vi "unpackAutonArray.vi"(0 "all rows":dbl[][](array[numeric])) -> (19 "ShootNow":dbl[](array[numeric]), 20 "Primitive":i16[](array[numeric]), 21 "Left Drive":dbl[](array[numeric]), 22 "Right Drive":dbl[](array[numeric]), 23 "Ramp ACT":dbl[](array[numeric]), 24 "Conveyor":dbl[](array[numeric]), 25 "Harvester":dbl[](array[numeric]), 26 "Turret":dbl[](array[numeric]), 27 "Shooter":dbl[](array[numeric]))   [LabVIEW 2011]
doc: "Use this VI to separate the autonomous array data into individual arrays. First array is Primitive ID, second is heading, etc."
panel:
  out "Misc 6":dbl[](array[numeric])
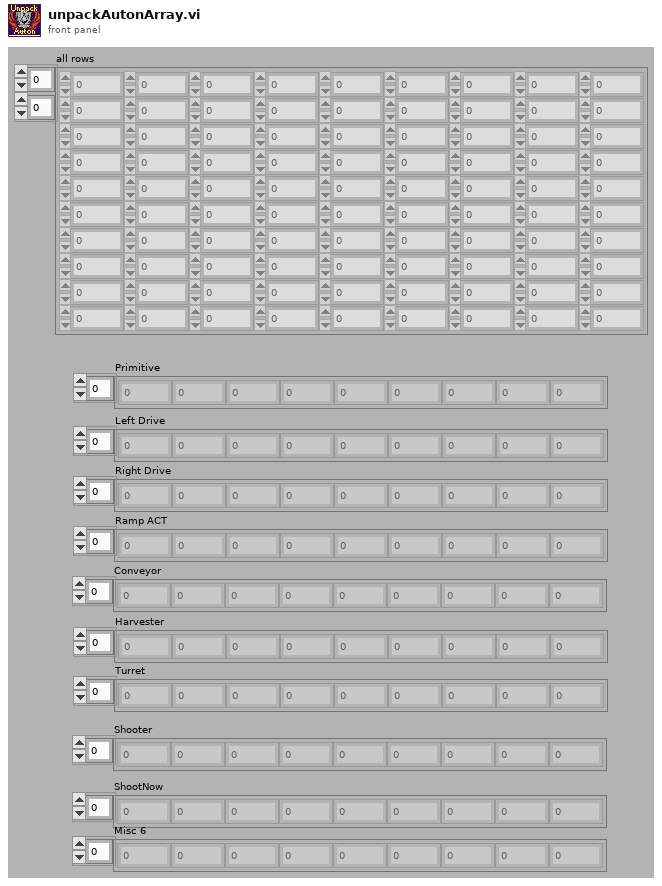
[diagram p1: front panel]
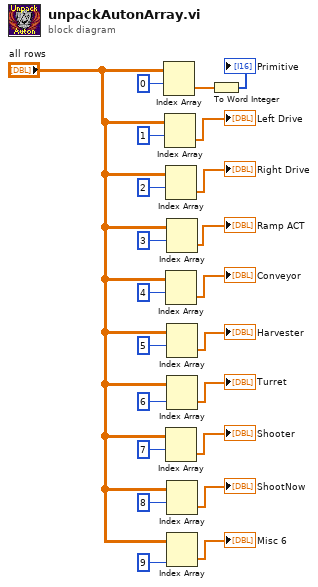
[diagram p0: block diagram]
diagram:
  n1 = Index Array(array="all rows", index (row)=0) -> (element=w19:dbl[])  [unwired: 1 in]
  n2 = Index Array(array="all rows", index (row)=1) -> (element=→"Left Drive":dbl[])  [unwired: 1 in]
  n3 = Index Array(array="all rows", index (row)=2) -> (element=→"Right Drive":dbl[])  [unwired: 1 in]
  n4 = Index Array(array="all rows", index (row)=4) -> (element=→"Conveyor":dbl[])  [unwired: 1 in]
  n5 = Index Array(array="all rows", index (row)=7) -> (element=→"Shooter":dbl[])  [unwired: 1 in]
  n6 = Index Array(array="all rows", index (row)=3) -> (element=→"Ramp ACT":dbl[])  [unwired: 1 in]
  n7 = Index Array(array="all rows", index (row)=5) -> (element=→"Harvester":dbl[])  [unwired: 1 in]
  n8 = Index Array(array="all rows", index (row)=6) -> (element=→"Turret":dbl[])  [unwired: 1 in]
  n9 = Index Array(array="all rows", index (row)=8) -> (element=→"ShootNow":dbl[])  [unwired: 1 in]
  n10 = Index Array(array="all rows", index (row)=9) -> (element=→"Misc 6":dbl[])  [unwired: 1 in]
  n11 = To Word Integer(number=w19) -> (16bit integer=→"Primitive":i16[])
